vi "Historical Data Access Client.vi"() -> ()   [LabVIEW 2019, in "OPC UA Demo.lvlib"]
doc: "Demonstrates the use of the <B>OPC UA Historical Data Access</B> functionality as an OPC UA Client."
uses:
  OPC UA Demo.lvlib
  <vilib>/OPCUA/client/Multiple Read Variant.vi
  <vilib>/OPCUA/NI OPC UA Client.lvlib
panel:
  out "Array":dbl[](array[numeric])
  in  "stop update":bool
  in  "start":bool
  in  "update type":enum32{"single update", "cyclic update"}(radio)
  in  "update interval":dbl=1.0 format="%<%H:%M:%S>t"
  in  "start time":timestamp
  in  "end time":timestamp
  in  "time span":dbl=3600.0 format="%<%H:%M:%S>t"
  out "historical data":cluster{cluster{"timestamp":timestamp, dbl}[]}[](graph)
  in  "update":bool
  in  "node ID":i32(listbox)
  in  "stop":bool
  in  "server endpoint URL":string="opc.tcp://localhost:49580"
  # "Overview: Demonstrates the use of the OPC UA Historical Data Access functionality as an OPC UA Client.\nRequirements: \n1. LabVIEW OPC UA Toolkit\n2. Run this VI on RT targets or Windows\nInstructions:\n1. Specify the server endpoint URL generated by the server.\n2. Run the VI.\n3. Choose single update or cyclic update to change the read mode of historical data."
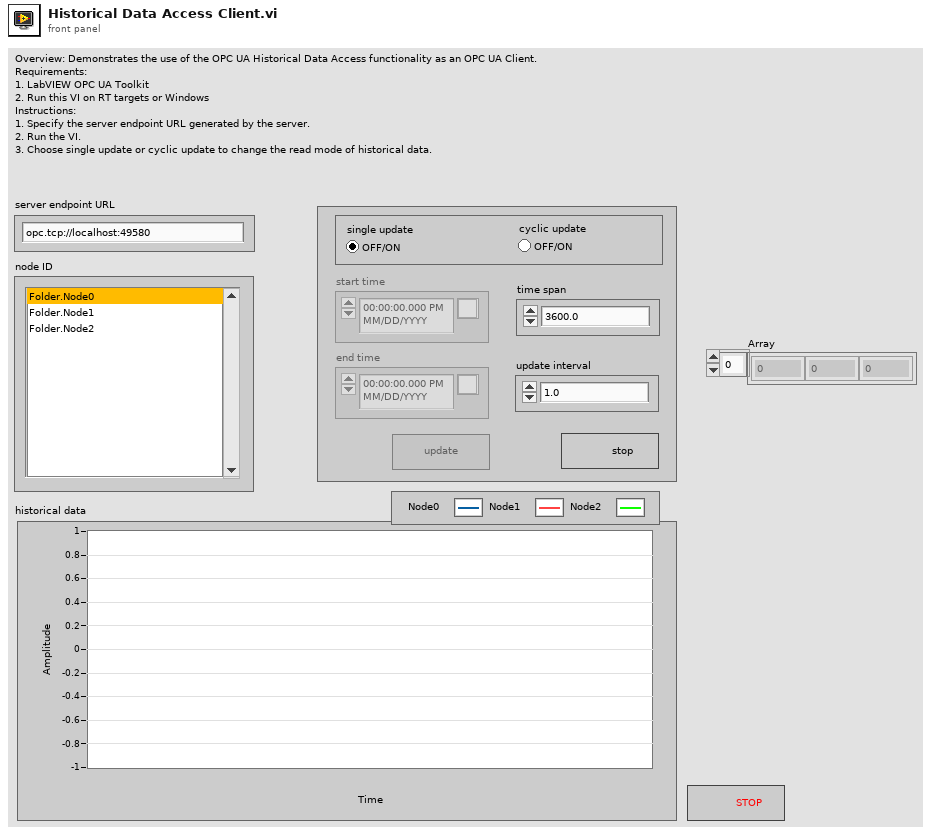
[diagram p1: front panel]
types:
  T1 = enum16{"Idle", "Initialize", "UpdateStart", "UpdateEnd", "Wait", "Stop"}
  T2 = enum8{"Enabled", "Disabled", "Disabled and Grayed Out"}
  T3 = cluster{"start time":timestamp, "end time":timestamp, "num values per node":u32, "return bounds":bool}
  T4 = typedef "OPC UA Client Refnum.ctl" = refnum<k21>
  T5 = typedef "Read Variant Result.ctl" = cluster{"node ID":T6, "value ":variant, "timestamp":timestamp, "status":T7}
  T6 = typedef "NodeId.ctl" = string
  T7 = typedef "OPC UA StatusCode.ctl" = u32
  T8 = typedef "History Data Result.ctl" = cluster{"node ID":T6, "history data":T9[], "status":T7}
  T9 = typedef "History Data.ctl" = cluster{"value ":variant, "timestamp":timestamp, "node status":T7}
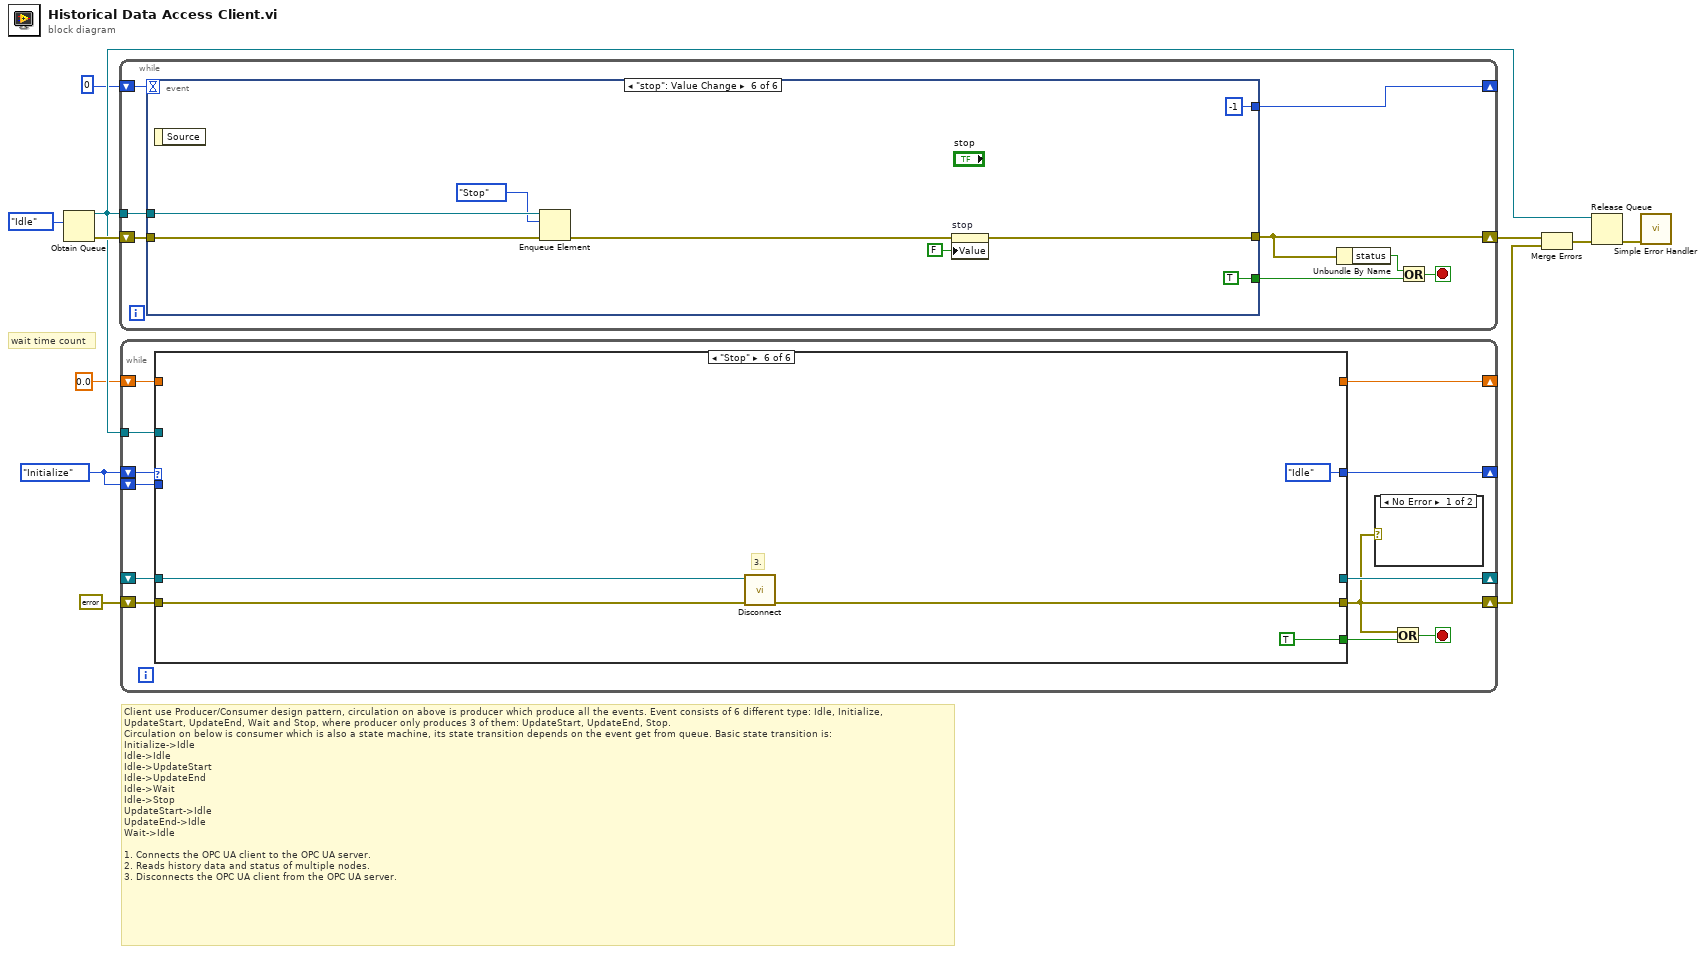
[diagram p0: block diagram]
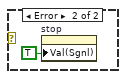
[diagram p2: hidden frame]
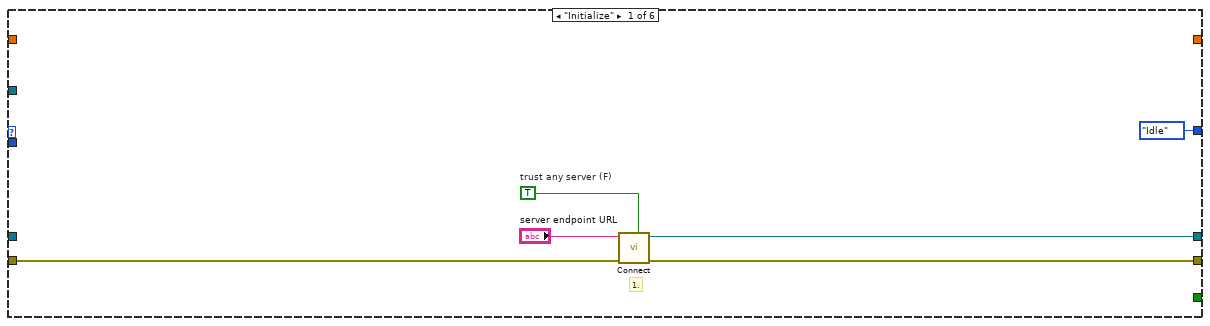
[diagram p3: hidden frame]
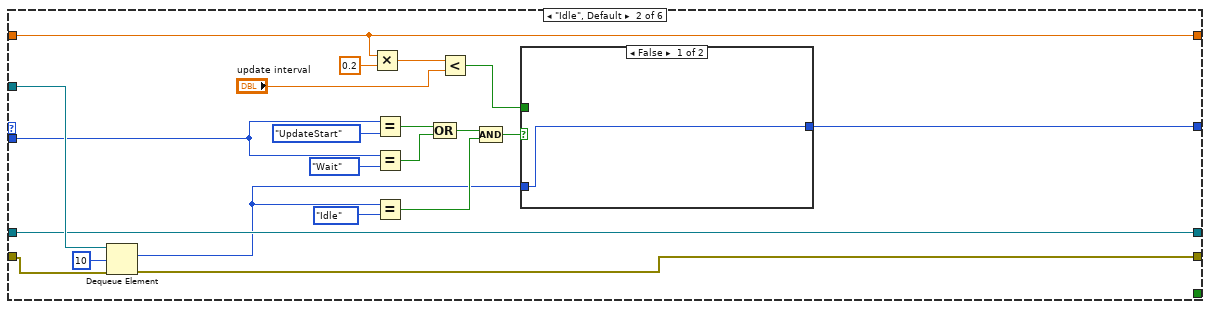
[diagram p4: hidden frame]
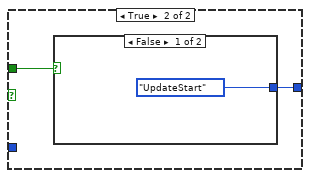
[diagram p5: hidden frame]
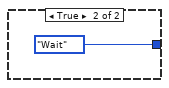
[diagram p6: hidden frame]
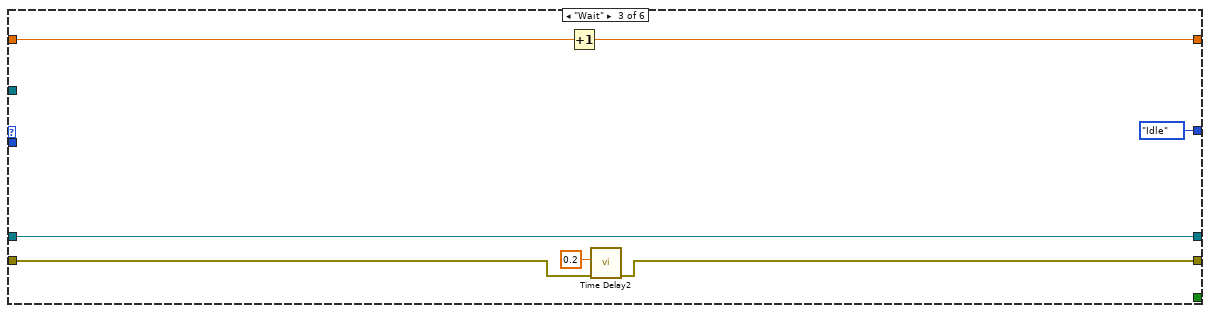
[diagram p7: hidden frame]
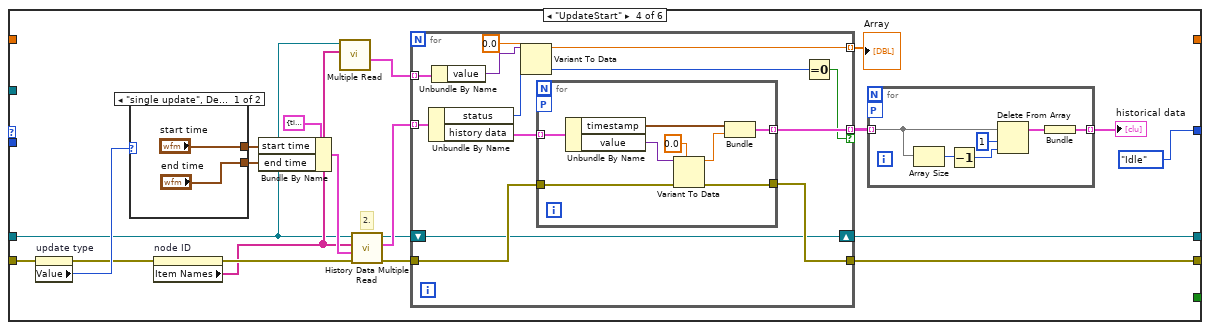
[diagram p8: hidden frame]
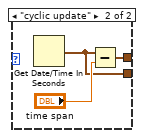
[diagram p9: hidden frame]
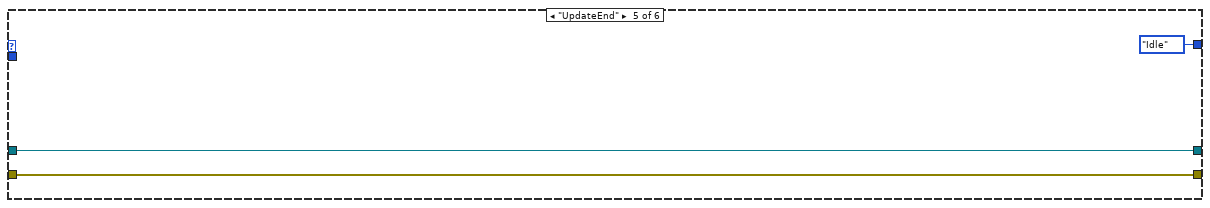
[diagram p10: hidden frame]
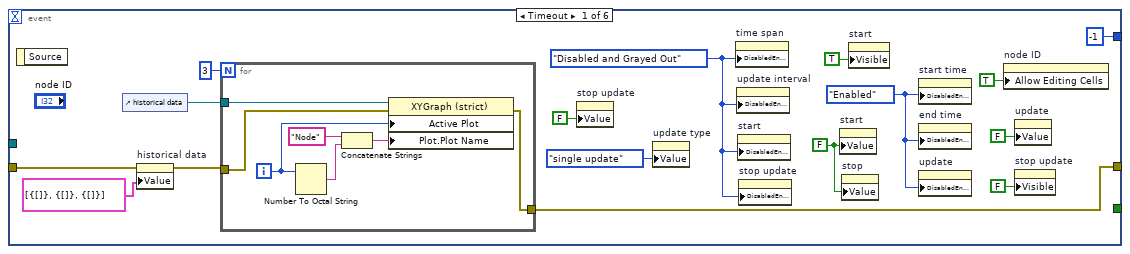
[diagram p11: hidden frame]
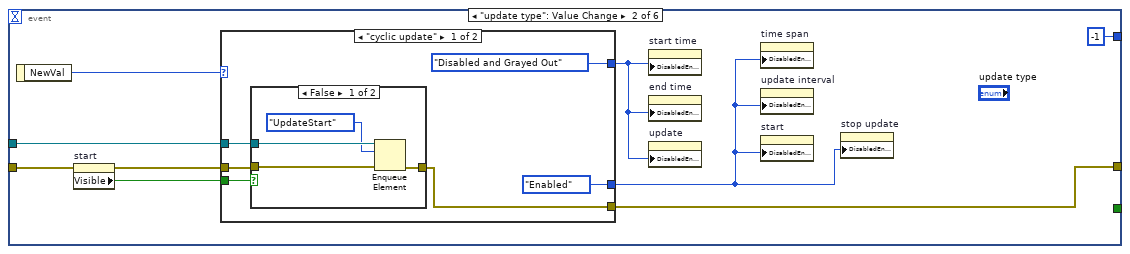
[diagram p12: hidden frame]
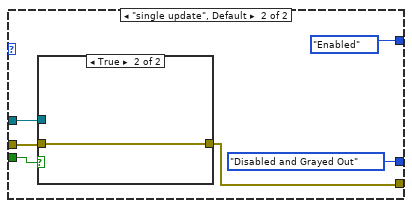
[diagram p14: hidden frame]
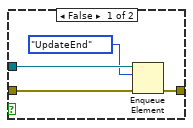
[diagram p15: hidden frame]
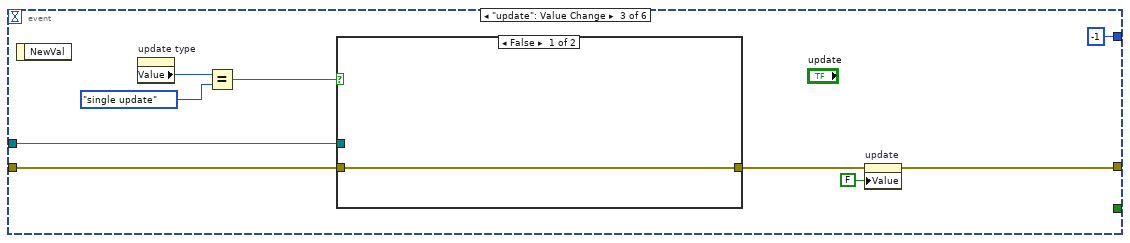
[diagram p16: hidden frame]
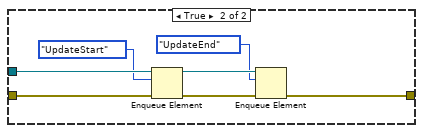
[diagram p17: hidden frame]
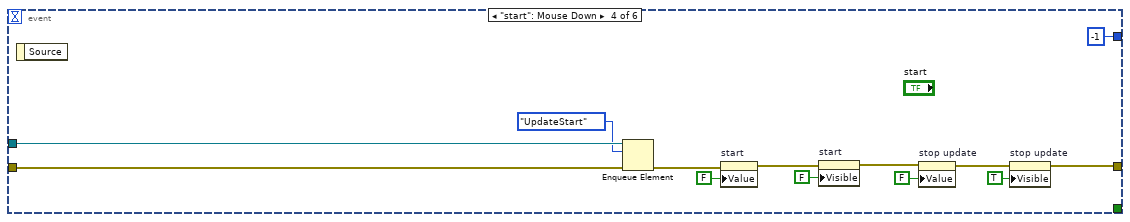
[diagram p18: hidden frame]
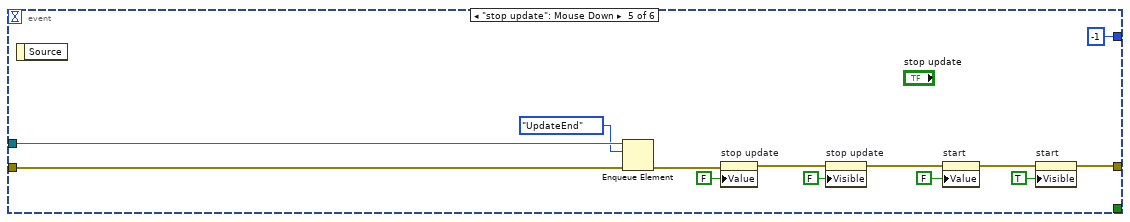
[diagram p19: hidden frame]
diagram:
  w1 = T1."Initialize"
  # "wait time count"
  # "Client use Producer/Consumer design pattern, circulation on above is producer which produce all the events. Event consists of 6 different type: Idle, Initialize, \nUpdateStart, UpdateEnd, Wait and Stop, where producer only produces 3 of them: UpdateStart, UpdateEnd, Stop.\nCirculation on below is consumer which is also a state machine, its state transition depends on the event get from queue. Basic state transition is: \nInitialize->Idle\nIdle->Idle\nIdle->UpdateStart\nIdle->UpdateEnd\nIdle->Wait\nIdle->Stop\nUpdateStart->Idle\nUpdateEnd->Idle\nWait->Idle\n\n1. Connects the OPC UA client to the OPC UA server.\n2. Reads history data and status of multiple nodes.\n3. Disconnects the OPC UA client from the OPC UA server."
  n1 = Obtain Queue(element data type=T1."Idle") -> (queue out=w10:refnum<queue>, error out=w11:errorcluster)  [unwired: 4 in, 1 out]
  n2 = while {
    shift-right: [w15] -> w8
    shift-left: w11 -> [w18]
    tunnel: w10 -> [w19]
    shift-right: [w12] -> _
    shift-left: 0 -> [w13]
    stop <- w16 stop-if-true
    n3 = event shown="[5] \"stop\": Value Change" {
      selector: _ -> [_ _ _ _ _ _]
      dyn-events: _ -> [_ _ _ _ _ _]
      timeout: w13 -> [_ _ _ _ _ _]
      tunnel: w19 -> [_ w45 w80 w103 w116 w121]
      tunnel: w18 -> [w28 w48 w79 w101 w114 w122]
      tunnel: [w22 w49 w76 w96 w108 w119] -> w15
      tunnel: [_ _ _ _ _ TRUE ("stop")] -> w17
      tunnel: [-1 -1 -1 -1 -1 -1] -> w12
      event Timeout {
        w27 = FALSE ("start")
        w31 = T2."Enabled" ("Disabled")
        w23 = T2."Disabled and Grayed Out" ("Disabled")
        n4 = event-data() -> ()  [unwired: 1 in, 1 out]
        n5 = control-ref of="historical data"() -> (w34:refnum<vi>)
        n6 = property on="historical data" class="XYGraph (strict)"(error in=w28, "Value"=cluster{cluster{"timestamp":timestamp, dbl}[]}[] [{[]}, {[]}, {[]}] ("history data")) -> (error out=w32:errorcluster)  [unwired: 1 in, 1 out]
        n7 = for {
          N: 3 -> [_]
          tunnel: w34 -> [w38]
          tunnel: w32 -> [w37]
          tunnel: [w36] -> w22
          i -> [w42]
          n8 = Number To Octal String(2:w42) -> (0:w40:string)  [unwired: 1 in]
          n9 = Concatenate Strings("Node" ("Plot.Plot Name"), w40) -> (w39:string)
          n10 = property class="XYGraph (strict)"(reference=w38, error in=w37, "Active Plot"=w42, "Plot.Plot Name"=w39) -> (error out=w36:errorcluster)  [unwired: 1 out]
        }
        n11 = property on="stop update" class="Bool (strict)"("Value"=FALSE ("stop update")) -> ()  [unwired: 2 in, 2 out]
        n12 = property on="update type" class="RadioBtnsControl (strict)"("Value"=enum32{"single update", "cyclic update"}."single update" ("update type")) -> ()  [unwired: 2 in, 2 out]
        n13 = property on="time span" class="DigNum (strict)"("DisabledEnum"=w23) -> ()  [unwired: 2 in, 2 out]
        n14 = property on="update interval" class="DigNum (strict)"("DisabledEnum"=w23) -> ()  [unwired: 2 in, 2 out]
        n15 = property on="start" class="Bool (strict)"("DisabledEnum"=w23) -> ()  [unwired: 2 in, 2 out]
        n16 = property on="stop update" class="Bool (strict)"("DisabledEnum"=w23) -> ()  [unwired: 2 in, 2 out]
        n17 = property on="start" class="Bool (strict)"("Value"=w27) -> ()  [unwired: 2 in, 2 out]
        n18 = property on="stop" class="Bool (strict)"("Value"=w27) -> ()  [unwired: 2 in, 2 out]
        n19 = property on="start" class="Bool (strict)"("Visible"=TRUE) -> ()  [unwired: 2 in, 2 out]
        n20 = property on="start time" class="AbsTime (strict)"("DisabledEnum"=w31) -> ()  [unwired: 2 in, 2 out]
        n21 = property on="end time" class="AbsTime (strict)"("DisabledEnum"=w31) -> ()  [unwired: 2 in, 2 out]
        n22 = property on="update" class="Bool (strict)"("DisabledEnum"=w31) -> ()  [unwired: 2 in, 2 out]
        n23 = property on="node ID" class="LstBox (strict)"("Allow Editing Cells"=TRUE) -> ()  [unwired: 2 in, 2 out]
        n24 = property on="update" class="Bool (strict)"("Value"=FALSE ("update")) -> ()  [unwired: 2 in, 2 out]
        n25 = property on="stop update" class="Bool (strict)"("Visible"=FALSE) -> ()  [unwired: 2 in, 2 out]
      }
      event "update type": Value Change {
        n26 = event-data() -> ("NewVal"=w51:enum32{"single update", "cyclic update"})  [unwired: 1 in]
        n27 = property on="start" class="Bool (strict)"(error in=w48) -> (error out=w47:errorcluster, "Visible"=w44:bool)  [unwired: 1 in, 1 out]
        n28 = case shown="\"cyclic update\"" w51 {
          tunnel: w47 -> [w55 w66]
          tunnel: w45 -> [w57 w68]
          tunnel: [w56 w67] -> w49
          tunnel: w44 -> [w54 w65]
          tunnel: [T2."Enabled" ("Disabled") T2."Disabled and Grayed Out" ("Disabled")] -> w43
          tunnel: [T2."Disabled and Grayed Out" ("Disabled") T2."Enabled" ("Disabled")] -> w46
          frame "cyclic update" {
            n29 = case shown="False" w54 {
              tunnel: w55 -> [w61 w62]
              tunnel: w57 -> [w59 _]
              tunnel: [w60 w62] -> w56
              frame False {
                n30 = Enqueue Element(queue=w59, element=T1."UpdateStart", error in (no error)=w61) -> (error out=w60:errorcluster)  [unwired: 1 in, 2 out]
              }
              frame True {
              }
            }
          }
          frame "single update", Default {
            n31 = case shown="True" w65 {
              tunnel: w66 -> [w72 w73]
              tunnel: w68 -> [w71 _]
              tunnel: [w70 w73] -> w67
              frame False {
                n32 = Enqueue Element(queue=w71, element=T1."UpdateEnd", error in (no error)=w72) -> (error out=w70:errorcluster)  [unwired: 1 in, 2 out]
              }
              frame True {
              }
            }
          }
        }
        n33 = property on="start time" class="AbsTime (strict)"("DisabledEnum"=w46) -> ()  [unwired: 2 in, 2 out]
        n34 = property on="end time" class="AbsTime (strict)"("DisabledEnum"=w46) -> ()  [unwired: 2 in, 2 out]
        n35 = property on="update" class="Bool (strict)"("DisabledEnum"=w46) -> ()  [unwired: 2 in, 2 out]
        n36 = property on="time span" class="DigNum (strict)"("DisabledEnum"=w43) -> ()  [unwired: 2 in, 2 out]
        n37 = property on="update interval" class="DigNum (strict)"("DisabledEnum"=w43) -> ()  [unwired: 2 in, 2 out]
        n38 = property on="start" class="Bool (strict)"("DisabledEnum"=w43) -> ()  [unwired: 2 in, 2 out]
        n39 = property on="stop update" class="Bool (strict)"("DisabledEnum"=w43) -> ()  [unwired: 2 in, 2 out]
      }
      event "update": Value Change {
        n40 = event-data() -> ()  [unwired: 1 in, 1 out]
        n41 = property on="update type" class="RadioBtnsControl (strict)"() -> ("Value"=w82:enum32{"single update", "cyclic update"})  [unwired: 2 in, 2 out]
        n42 = Equal?(x=w82, y=enum32{"single update", "cyclic update"}."single update") -> (x = y?=w81:bool)
        n43 = case shown="False" w81 {
          tunnel: w80 -> [_ w89]
          tunnel: w79 -> [w83 w90]
          tunnel: [w83 w86] -> w77
          frame False {
          }
          frame True {
            n44 = Enqueue Element(queue=w89, element=T1."UpdateStart", error in (no error)=w90) -> (queue out=w87:refnum<queue>, error out=w88:errorcluster)  [unwired: 1 in, 1 out]
            n45 = Enqueue Element(queue=w87, element=T1."UpdateEnd", error in (no error)=w88) -> (error out=w86:errorcluster)  [unwired: 1 in, 2 out]
          }
        }
        n46 = property on="update" class="Bool (strict)"(error in=w77, "Value"=FALSE ("update")) -> (error out=w76:errorcluster)  [unwired: 1 in, 1 out]
      }
      event "start": Mouse Down {
        n47 = event-data() -> ()  [unwired: 1 in, 1 out]
        n48 = Enqueue Element(queue=w103, element=T1."UpdateStart", error in (no error)=w101) -> (error out=w100:errorcluster)  [unwired: 1 in, 2 out]
        n49 = property on="start" class="Bool (strict)"(error in=w100, "Value"=FALSE ("start")) -> (error out=w98:errorcluster)  [unwired: 1 in, 1 out]
        n50 = property on="start" class="Bool (strict)"(error in=w98, "Visible"=FALSE) -> (error out=w93:errorcluster)  [unwired: 1 in, 1 out]
        n51 = property on="stop update" class="Bool (strict)"(error in=w93, "Value"=FALSE ("stop update")) -> (error out=w92:errorcluster)  [unwired: 1 in, 1 out]
        n52 = property on="stop update" class="Bool (strict)"(error in=w92, "Visible"=TRUE ("stop update")) -> (error out=w96:errorcluster)  [unwired: 1 in, 1 out]
      }
      event "stop update": Mouse Down {
        n53 = event-data() -> ()  [unwired: 1 in, 1 out]
        n54 = Enqueue Element(queue=w116, element=T1."UpdateEnd", error in (no error)=w114) -> (error out=w113:errorcluster)  [unwired: 1 in, 2 out]
        n55 = property on="stop update" class="Bool (strict)"(error in=w113, "Value"=FALSE ("start")) -> (error out=w109:errorcluster)  [unwired: 1 in, 1 out]
        n56 = property on="stop update" class="Bool (strict)"(error in=w109, "Visible"=FALSE ("stop update")) -> (error out=w107:errorcluster)  [unwired: 1 in, 1 out]
        n57 = property on="start" class="Bool (strict)"(error in=w107, "Value"=FALSE ("Visible")) -> (error out=w106:errorcluster)  [unwired: 1 in, 1 out]
        n58 = property on="start" class="Bool (strict)"(error in=w106, "Visible"=TRUE) -> (error out=w108:errorcluster)  [unwired: 1 in, 1 out]
      }
      event "stop": Value Change {
        n59 = event-data() -> ()  [unwired: 1 in, 1 out]
        n60 = Enqueue Element(queue=w121, element=T1."Stop", error in (no error)=w122) -> (error out=w120:errorcluster)  [unwired: 1 in, 2 out]
        n61 = property on="stop" class="Bool (strict)"(error in=w120, "Value"=FALSE ("stop")) -> (error out=w119:errorcluster)  [unwired: 1 in, 1 out]
      }
    }
    n62 = Unbundle By Name(w15) -> ("status"=w14:bool)
    n63 = Or(x=w14, y=w17) -> (x .or. y?=w16:bool)
  }
  n64 = while {
    tunnel: w10 -> [w128]
    shift-right: [w136] -> _
    shift-left: _ -> [w135]
    shift-right: [w132] -> w5
    shift-left: errorcluster {"status"=FALSE, "code"=0, "source"=""} ("error out") -> [w129]
    shift-right: [w125] -> _
    shift-left: w1 -> [w131]
    shift-left: w1 -> [w130]
    shift-right: [w126] -> _
    shift-left: 0.0 -> [w127]
    stop <- w133 stop-if-true
    n65 = case shown="\"Stop\"" w131 {
      tunnel: w129 -> [w139 w150 w171 w195 w229 w234]
      tunnel: [_ _ _ _ _ TRUE] -> w134
      tunnel: [w142 w149 w172 w183 w230 _] -> w136
      tunnel: w135 -> [_ w149 w172 w179 w230 w235]
      tunnel: [T1."Idle" w163 T1."Idle" T1."Idle" T1."Idle" T1."Idle"] -> w125
      tunnel: [w141 w158 w175 w184 w229 w233] -> w132
      tunnel: w130 -> [_ w148 _ _ _ _]
      tunnel: w128 -> [_ w161 _ _ _ _]
      tunnel: w127 -> [_ w144 w174 _ _ _]
      tunnel: [_ w144 w173 _ _ _] -> w126
      frame "Initialize" {
        w138 = TRUE  # trust any server (F)
        # "1."
        n66 = call <vilib>:"Connect.vi"("trust any server (F)"=w138, "error in (no error)"=w139, "server endpoint URL"="server endpoint URL") -> ("error out"=w141:errorcluster, "OPC UA client refnum out"=w142:T4)  [unwired: 6 in, 1 out]
      }
      frame "Idle", Default {
        n67 = Dequeue Element(queue=w161, timeout in ms (-1)=10, error in (no error)=w150) -> (element=w145:T1, error out=w158:errorcluster)  [unwired: 2 out]
        n68 = Multiply(x=w144, y=0.2) -> (x*y=w156:dbl)
        n69 = Equal?(x=w148, y=T1."UpdateStart") -> (x = y?=w153:bool)
        n70 = Equal?(x=w148, y=T1."Wait") -> (x = y?=w152:bool)
        n71 = Equal?(x=w145, y=T1."Idle") -> (x = y?=w146:bool)
        n72 = Compound Arithmetic op=OR(w153, w152) -> (w147:bool)
        n73 = Less?(x=w156, y="update interval") -> (x < y?=w151:bool)
        n74 = Compound Arithmetic op=AND(w147, w146) -> (w164:bool)
        n75 = case shown="False" w164 {
          tunnel: [w165 w167] -> w163
          tunnel: w151 -> [_ w166]
          tunnel: w145 -> [w165 _]
          frame False {
          }
          frame True {
            n76 = case shown="False" w166 {
              tunnel: [T1."UpdateStart" T1."Wait"] -> w167
              frame False {
              }
              frame True {
              }
            }
          }
        }
      }
      frame "Wait" {
        n77 = Increment(x=w174) -> (x+1=w173:dbl)
        n78 = call "Time Delay2"("error in (no error)"=w171, "Delay Time (s)"=0.2) -> ("error out"=w175:errorcluster)  [unwired: 9 in]
      }
      frame "UpdateStart" {
        # "2."
        n79 = property on="update type" class="RadioBtnsControl (strict)"(error in=w195) -> (error out=w191:errorcluster, "Value"=w196:enum32{"single update", "cyclic update"})  [unwired: 1 in, 1 out]
        n80 = case shown="\"single update\", Default" w196 {
          tunnel: ["start time" w226] -> w194
          tunnel: ["end time" w225] -> w193
          frame "single update", Default {
          }
          frame "cyclic update" {
            n81 = Get Date/Time In Seconds() -> (seconds since 1Jan1904=w225:timestamp)
            n82 = Subtract(x=w225, y="time span") -> (x-y=w226:timestamp)
          }
        }
        n83 = property on="node ID" class="LstBox (strict)"(error in=w191) -> (error out=w190:errorcluster, "Item Names"=w180:string[])  [unwired: 1 in, 1 out]
        n84 = Bundle By Name(cluster=T3 {"start time"=timestamp(0 s since 1904-01-01), "end time"=timestamp(0 s since 1904-01-01), "num values per node"=0, "return bounds"=FALSE} ("request"), "start time"=w194, "end time"=w193) -> (w192:T3)
        n85 = call-poly <vilib>:"Multiple Read.vi"("node IDs"=w180, "OPC UA client refnum in"=w179) -> ("results"=w178:T5[])  [unwired: 6 in, 3 out]
        n86 = call <vilib>:"History Data Multiple Read.vi"("error in (no error)"=w190, "request"=w192, "node IDs"=w180, "OPC UA client refnum in"=w179) -> ("error out"=w185:errorcluster, "results"=w188:T8[], "OPC UA client refnum out"=w186:T4)  [unwired: 3 in, 2 out]
        n87 = for {
          tunnel: [w208] -> w187 mode=indexing if=w204
          tunnel: w188 -> [w206] mode=indexing
          tunnel: w185 -> [w203]
          tunnel: [w202] -> w184
          shift-right: [w201] -> w183
          shift-left: w186 -> [w201]
          tunnel: w178 -> [w200] mode=indexing
          tunnel: [w197] -> w177 mode=indexing
          n88 = Unbundle By Name(w206) -> ("status"=w205:T7, "history data"=w207:T9[])
          n89 = Unbundle By Name(w200) -> ("value"=w198:variant)
          n90 = Variant To Data(type=0.0, Variant=w198) -> (data=w197:dbl)  [unwired: 1 in, 1 out]
          n91 = for {
            tunnel: w207 -> [w216] mode=indexing
            tunnel: [w215] -> w208 mode=indexing
            tunnel: w203 -> [w210]
            tunnel: [w209] -> w202
            workers-P: _ -> [_]
            n92 = Unbundle By Name(w216) -> ("timestamp"=w212:timestamp, "value"=w211:variant)
            n93 = Variant To Data(error in=w210, type=0.0, Variant=w211) -> (data=w213:dbl, error out=w209:errorcluster)
            n94 = Bundle("timestamp"=w212, w213) -> (w215:cluster{"timestamp":timestamp, dbl})  [unwired: 1 in]
          }
          n95 = Equal To 0?(x=w205) -> (x = 0?=w204:bool)
        }
        "Array" <- w177
        n96 = for {
          tunnel: w187 -> [w220] mode=indexing
          tunnel: [w222] -> w182 mode=indexing
          workers-P: _ -> [_]
          n97 = Array Size(array=w220) -> (size(s)=w221:i32)
          n98 = Decrement(x=w221) -> (x-1=w218:i32)
          n99 = Delete From Array(array=w220, length=1, index=w218) -> (array with subset deleted=w217:cluster{"timestamp":timestamp, dbl}[])  [unwired: 1 out]
          n100 = Bundle(w217) -> (w222:cluster{cluster{"timestamp":timestamp, dbl}[]})  [unwired: 1 in]
        }
        "historical data" <- w182
      }
      frame "UpdateEnd" {
      }
      frame "Stop" {
        # "3."
        n101 = call <vilib>:"Disconnect.vi"("error in (no error)"=w234, "OPC UA client refnum in"=w235) -> ("error out"=w233:errorcluster)  [unwired: 9 in]
      }
    }
    n102 = case shown="No Error" w132 {
      frame No Error {
      }
      frame Error {
        n103 = property on="stop" class="Bool (strict)"("Val(Sgnl)"=TRUE ("stop")) -> ()  [unwired: 2 in, 2 out]
      }
    }
    n104 = Or(x=w132, y=w134) -> (x .or. y?=w133:bool)
  }
  n105 = Merge Errors(w8, w5) -> (w7:errorcluster)
  n106 = Release Queue(queue=w10, error in (no error)=w7) -> (error out=w6:errorcluster)  [unwired: 1 in, 2 out]
  n107 = call <vilib>:"Simple Error Handler.vi"("error in (no error)"=w6) -> ()  [unwired: 4 in, 5 out]
